vi "Phase.vi"(2 "v Ctrl in":refnum<class "CtrlLine.lvclass">, 7 "QuWire in":refnum<class "QuWire.lvclass">, 11 "phi":dbl, 13 "^ Ctrl in":refnum<class "CtrlLine.lvclass">) -> (8 "QuWire out":refnum<class "QuWire.lvclass">)   [LabVIEW 2020]
doc: "Phase Gate (P)\n\nApplies an arbitrary phase shift phi to the |1> state. Leaves the |0> state unchanged. This corresponds to a rotation around the Z-axis by phi (relative to the global phase).\nPhase Gate (P) is a generalization of the Z, S, and T gates.\n\nMatrix: [[ 1, 0], [ 0, exp(i*phi) ]]"
uses:
  QuSim/QuWire/QuWire.lvclass
  QuSim/QuWire/CtrlLine/CtrlLine.lvclass
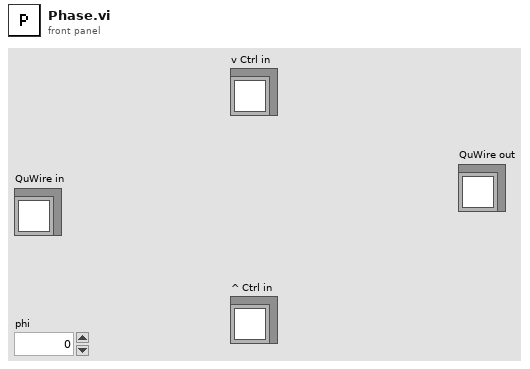
[diagram p1: front panel]
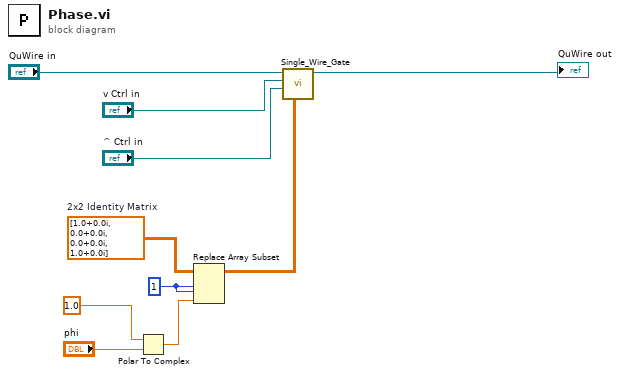
[diagram p0: block diagram]
diagram:
  w4 = 1 ("index (row)")
  w3 = cdb[][] [[1.0+0.0i, 0.0+0.0i], [0.0+0.0i, 1.0+0.0i]]  # 2x2 Identity Matrix
  n1 = Polar To Complex(1:"phi", 2:1.0 ("r")) -> (0:w6:cdb)
  n2 = Replace Array Subset(array=w3, new element=w6, index (row)=w4, index (col)=w4) -> (w1:cdb[][])
  n3 = call "Single_Wire_Gate.vi"("2x2 Unitary Matrix"=w1, "d CtrlLine in"="^ Ctrl in", "u CtrlLine in"="v Ctrl in", "QuWire in"="QuWire in") -> ("QuWire out"=→"QuWire out":refnum<class "QuWire.lvclass">)  [unwired: 6 in, 1 out]
